vi "Check Status (No Objects) - Spectrometer.vi"(8 "error in (no error)":errorcluster, 10 "VISA Resource Name":refnum<visa-resource-name>="GPIB0::1::INSTR", 11 "Cluster In":T4) -> (0 "error out":errorcluster, 1 "Status":string, 2 "Ready?":bool, 3 "Cluster Out":T4)   [LabVIEW 2012]
doc: "Checks if the instrument is powered on and updates its member data with the instrument's current status."
uses:
  JY-SPEX-TRIAX/controls.llb/Monochromator System Number.ctl
  JY-SPEX-TRIAX/controls.llb/Mirror Position.ctl
  JY-SPEX-TRIAX/controls.llb/Turret Position (TRIAX).ctl
  JY-SPEX-TRIAX/controls.llb/Slits.ctl
  JY-SPEX-TRIAX/JY-SPEX-TRIAX.lvlib
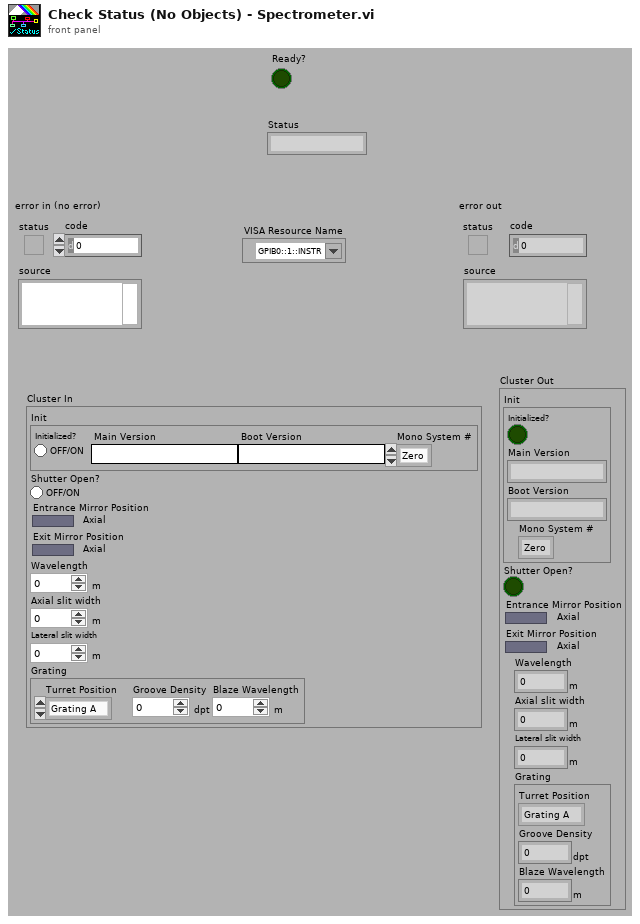
[diagram p1: front panel]
types:
  T1 = typedef "JY-SPEX-TRIAX.lvlib/Monochromator System Number.ctl" = enum16{"Zero", "One"}
  T2 = typedef "JY-SPEX-TRIAX.lvlib/Mirror Position.ctl" = bool
  T3 = typedef "JY-SPEX-TRIAX.lvlib/Turret Position (TRIAX).ctl" = enum16{"Grating A", "Grating B", "Grating C"}
  T4 = cluster{"Init":cluster{"Initialized?":bool, "Main Version":string, "Boot Version":string, "Mono System #":T1}, "Shutter Open?":bool, "Entrance Mirror Position":T2, "Exit Mirror Position":T2, "Wavelength":dbl[unit], "Axial slit width":dbl[unit], "Lateral slit width":dbl[unit], "Grating":cluster{"Turret Position":T3, "Groove Density":dbl[unit], "Blaze Wavelength":dbl[unit]}}
  T5 = typedef "JY-SPEX-TRIAX.lvlib/Slits.ctl" = enum16{"0 (Front/Axial Entrance)", "1 (Side/Lateral Entrance)", "2 (Front/Axial Exit)", "3 (Side/Lateral Exit)"}
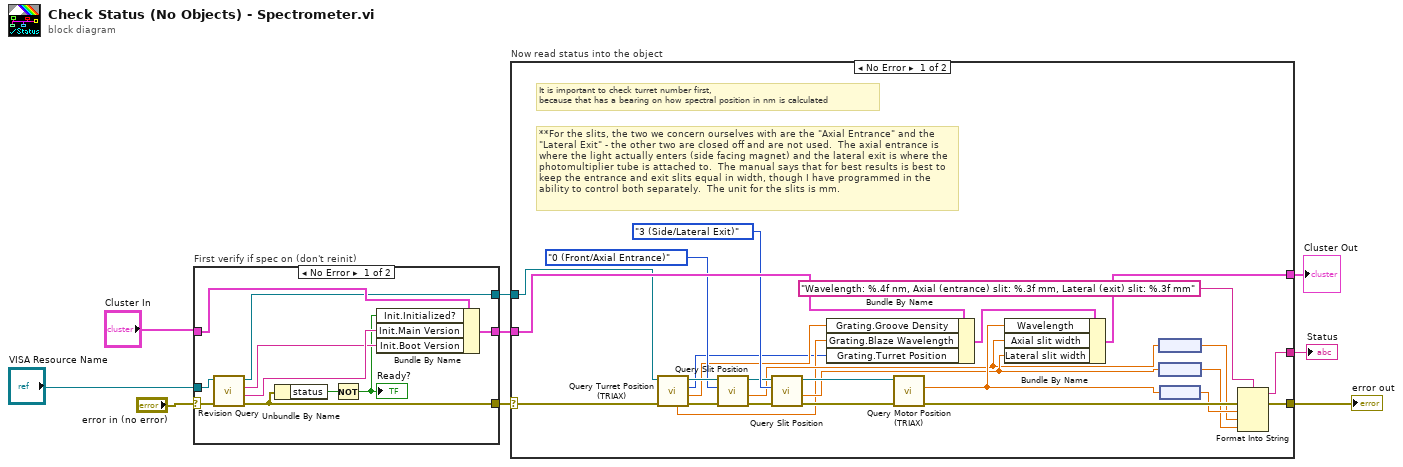
[diagram p0: block diagram]
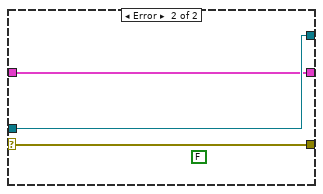
[diagram p2: hidden frame]
diagram:
  n1 = case "First verify if spec on (don't reinit)" shown="No Error" "error in (no error)" {
    selector: "error in (no error)" -> [w15 w22]
    tunnel: [w19 w20] -> w8
    tunnel: "Cluster In" -> [w18 w20]
    tunnel: "VISA Resource Name" -> [w17 w21]
    tunnel: [w16 w22] -> w7
    tunnel: [w13 w21] -> w6
    frame No Error {
      n2 = call "Revision Query.vi"("error in (no error)"=w15, "VISA resource name"=w17) -> ("error out"=w16:errorcluster, "Main Firmware Revision"=w12:string, "Boot Firmware Revision"=w11:string, "VISA resource name out"=w13:refnum<visa-resource-name>)  [unwired: 6 out]
      n3 = Unbundle By Name(w16) -> ("status"=w14:bool)
      n4 = Not(x=w14) -> (.not. x?=w10:bool)
      "Ready?" <- w10
      n5 = Bundle By Name(cluster=w18, "Init.Initialized?"=w10, "Init.Main Version"=w12, "Init.Boot Version"=w11) -> (w19:T4)
    }
    frame Error {
      (unwired) FALSE ("status")
    }
  }
  n6 = case "Now read status into the object" shown="No Error" w7 {
    selector: w7 -> [w29 w49]
    tunnel: w8 -> [w44 w50]
    tunnel: [w43 w50] -> w2
    tunnel: [w46 w49] -> w3
    tunnel: [w45 _] -> w9
    tunnel: w6 -> [w42 _]
    frame No Error {
      # "**For the slits, the two we concern ourselves with are the \"Axial Entrance\" and the \"Lateral Exit\" - the other two are closed off and are not used.  The axial entrance is where the light actually enters (side facing magnet) and the lateral exit is where the photomultiplier tube is attached to.  The manual says that for best results is best to keep the entrance and exit slits equal in width, though I have programmed in the ability to control both separately.  The unit for the slits is mm."
      # "It is important to check turret number first, \nbecause that has a bearing on how spectral position in nm is calculated"
      n7 = call "Query Turret Position (TRIAX).vi"("error in (no error)"=w29, "VISA resource name"=w42) -> ("error out"=w40:errorcluster, "Groove Density"=w28:dbl[unit], "Turret Position"=w26:T3, "VISA resource name out"=w41:refnum<visa-resource-name>, "Blaze Wavelength"=w27:dbl[unit])  [unwired: 1 in, 4 out]
      n8 = call "Query Slit Position.vi"("error in (no error)"=w40, "Slit (Front/Axial Entrance)"=Slits."0 (Front/Axial Entrance)", "VISA resource name"=w41) -> ("error out"=w37:errorcluster, "Slit Position"=w30:dbl[unit], "VISA resource name out"=w36:refnum<visa-resource-name>)  [unwired: 1 in, 5 out]
      n9 = call "Query Slit Position.vi"("error in (no error)"=w37, "Slit (Front/Axial Entrance)"=Slits."3 (Side/Lateral Exit)", "VISA resource name"=w36) -> ("error out"=w34:errorcluster, "Slit Position"=w31:dbl[unit], "VISA resource name out"=w35:refnum<visa-resource-name>)  [unwired: 1 in, 5 out]
      n10 = Bundle By Name(cluster=w44, "Grating.Groove Density"=w28, "Grating.Blaze Wavelength"=w27, "Grating.Turret Position"=w26) -> (w47:T4)
      n11 = call "Query Motor Position (TRIAX).vi"("error in (no error)"=w34, "VISA resource name"=w35) -> ("error out"=w33:errorcluster, "wavelength"=w32:dbl[unit])  [unwired: 1 in, 7 out]
      n12 = Bundle By Name(cluster=w47, "Wavelength"=w32, "Axial slit width"=w30, "Lateral slit width"=w31) -> (w43:T4)
      n13 = node(w30) -> (w24:dbl)
      n14 = node(w31) -> (w23:dbl)
      n15 = node(w32) -> (w25:dbl)
      n16 = Format Into String(format string="Wavelength: %.4f nm, Axial (entrance) slit: %.3f mm, Lateral (exit) slit: %.3f mm", error in=w33, w25, w24, w23) -> (resulting string=w45:string, error out=w46:errorcluster)  [unwired: 1 in]
    }
    frame Error {
    }
  }
  "error out" <- w3
  "Status" <- w9
  "Cluster Out" <- w2
